vi "LUnit Stop Test.vi"(8 "error in (no error)":errorcluster, 11 "Coverage Report in":refnum<class "Coverage Report.lvclass">) -> (0 "error out":errorcluster, 3 "Coverage Report out":refnum<class "Coverage Report.lvclass">)   [LabVIEW 2020, in "Coverage Report.lvclass"]
uses:
  Coverage Report.lvclass
  Coverage Report.lvclass/Coverage Report.ctl
  c80752a9-34a8-4590-82a2-f6539b8745c6.vi
  <vilib>/Platform/browser.llb/Open URL in Default Browser (path).vi
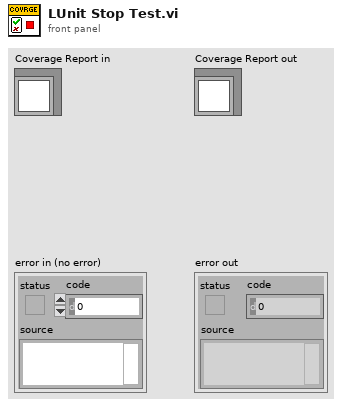
[diagram p1: front panel]
types:
  T1 = enum16{"open", "replace", "create", "open or create", "replace or create", "replace or create with confirmation"}
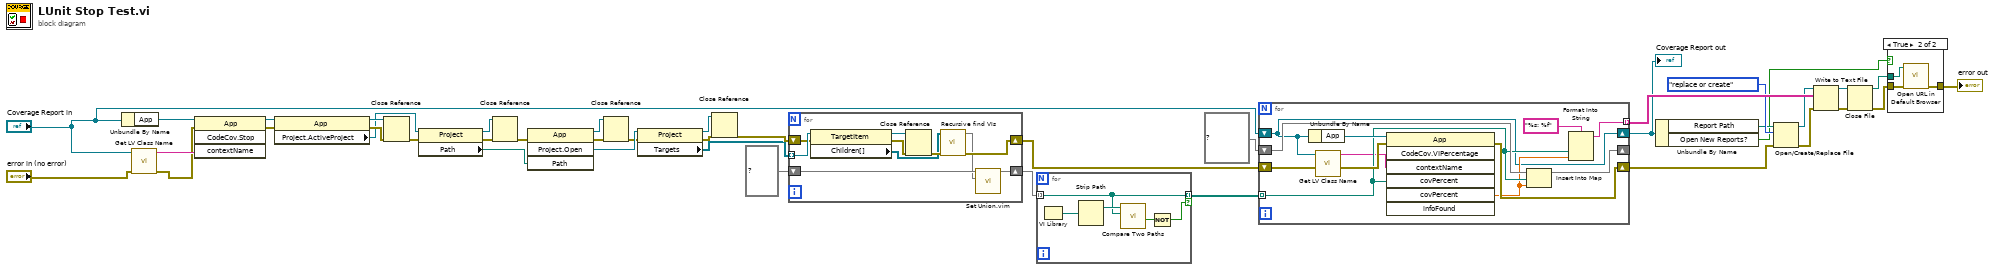
[diagram p0: block diagram]
diagram:
  n1 = Unbundle By Name("Coverage Report in") -> ("App"=w6:refnum<vi>)
  n2 = call <vilib>:"Get LV Class Name.vi"("error in (no error)"="error in (no error)", "object"="Coverage Report in") -> ("error out"=w1:errorcluster, "class name"=w3:string)  [unwired: 8 in]
  n3 = invoke class="App" method="CodeCov.Stop"(reference=w6, error in=w1, "contextName"=w3) -> (reference out=w13:refnum<vi>, error out=w16:errorcluster)  [unwired: 1 in, 2 out]
  n4 = property class="App"(reference=w13, error in=w16) -> (reference out=w8:refnum<vi>, error out=w11:errorcluster, "Project.ActiveProject"=w7:refnum<vi>)
  n5 = Close Reference(reference=w8, error in (no error)=w11) -> (error out=w12:errorcluster)
  n6 = property class="Project"(reference=w7, error in=w12) -> (reference out=w9:refnum<vi>, error out=w10:errorcluster, "Path"=w15:path)
  n7 = Close Reference(reference=w9, error in (no error)=w10) -> (error out=w17:errorcluster)
  n8 = invoke class="App" method="Project.Open"(error in=w17, "Path"=w15) -> (reference out=w22:refnum<vi>, error out=w26:errorcluster, "Project:Open"=w28:refnum<vi>)  [unwired: 2 in, 1 out]
  n9 = Close Reference(reference=w22, error in (no error)=w26) -> (error out=w23:errorcluster)
  n10 = property class="Project"(reference=w28, error in=w23) -> (reference out=w24:refnum<vi>, error out=w27:errorcluster, "Targets"=w19:refnum<vi>[])
  n11 = Close Reference(reference=w24, error in (no error)=w27) -> (error out=w25:errorcluster)
  n12 = for {
    tunnel: w19 -> [w51] mode=indexing
    shift-right: [w48] -> w14
    shift-left: w25 -> [w49]
    shift-right: [w44] -> w20
    shift-left: set{path} {} ("VIs") -> [w46]
    n13 = property class="TargetItem"(reference=w51, error in=w49) -> (reference out=w47:refnum<vi>, error out=w50:errorcluster, "Children[]"=w42:refnum<vi>[])
    n14 = Close Reference(reference=w47, error in (no error)=w50) -> (error out=w43:errorcluster)
    n15 = call "Recursive find VIs.vi"("error in (no error)"=w43, "Project Items"=w42) -> ("error out"=w48:errorcluster, "VIs"=w45:set{path})  [unwired: 8 in]
    n16 = call "Set Union.vim"("set 2"=w45, "set 1"=w46) -> ("union"=w44:set{path})  [unwired: 9 in]
  }
  n17 = for {
    tunnel: w20 -> [w54] mode=indexing
    tunnel: [w54] -> w29 mode=indexing if=w52
    n18 = VI Library() -> (path=w53:path)
    n19 = Strip Path(path=w53) -> (stripped path=w55:path)  [unwired: 1 out]
    n20 = call <vilib>:"Compare Two Paths.vi"("Path 2"=w54, "Path 1"=w55) -> ("Path 2 Relative to Path 1?"=w56:bool)  [unwired: 6 in, 3 out]
    n21 = Not(x=w56) -> (.not. x?=w52:bool)
  }
  n22 = for {
    shift-right: [w58] -> w5
    shift-left: "Coverage Report in" -> [w58]
    shift-right: [w66] -> w37
    shift-left: w14 -> [w67]
    tunnel: w29 -> [w61] mode=indexing
    shift-right: [w64] -> _
    shift-left: map{path, dbl} {} ("Code Coverage") -> [w65]
    tunnel: [w59] -> w39 mode=indexing
    n23 = Unbundle By Name(w58) -> ("App"=w63:refnum<vi>)
    n24 = call <vilib>:"Get LV Class Name.vi"("object"=w58) -> ("class name"=w57:string)  [unwired: 9 in, 1 out]
    n25 = invoke class="App" method="CodeCov.VIPercentage"(reference=w63, error in=w67, "contextName"=w57, "covPercent"=w61) -> (error out=w66:errorcluster, "covPercent"=w60:dbl)  [unwired: 3 in, 5 out]
    n26 = Insert Into Map(map in=w65, key=w61, value=w60) -> (map out=w64:map{path, dbl})  [unwired: 2 out]
    n27 = Format Into String(format string="%s: %f", w61, w60) -> (resulting string=w59:string)  [unwired: 2 in, 1 out]
  }
  "Coverage Report out" <- w5
  n28 = Unbundle By Name(w5) -> ("Report Path"=w35:path, "Open New Reports?"=w30:bool)
  n29 = Open/Create/Replace File(file path (use dialog)=w35, error in=w37, operation (0:open)=T1."replace or create") -> (refnum out=w31:refnum<file>, error out=w32:errorcluster)  [unwired: 3 in, 1 out]
  n30 = Write to Text File(file (use dialog)=w31, text=w39, error in=w32) -> (refnum out=w33:refnum<file>, error out=w34:errorcluster)  [unwired: 1 in, 1 out]
  n31 = Close File(refnum=w33, error in=w34) -> (path=w41:path, error out=w36:errorcluster)
  n32 = case shown="True" w30 {
    tunnel: w41 -> [_ w69]
    tunnel: w36 -> [w68 w71]
    tunnel: [w68 w70] -> w40
    frame False {
    }
    frame True {
      n33 = call-poly <vilib>:"Open URL in Default Browser.vi"("error in (no error)"=w71, "path"=w69) -> ("error out"=w70:errorcluster)  [unwired: 4 in, 1 out]
    }
  }
  "error out" <- w40
